vi "TypeDescriptor_ListElementNames.vi"(11 "type descriptor":i16[](array[numeric]) format="%04x") -> (1 "Has Elements":bool, 2 "element names":string[](array[string]), 3 "type descriptor dup":i16[](array[numeric]) format="%.0x", 4 "Event Class":string[](array[string]))   [LabVIEW 2013, in "OpenDescriptor.lvlib"]
uses:
  OpenDescriptor.lvlib
  TypeDescriptor_GetPString.vi
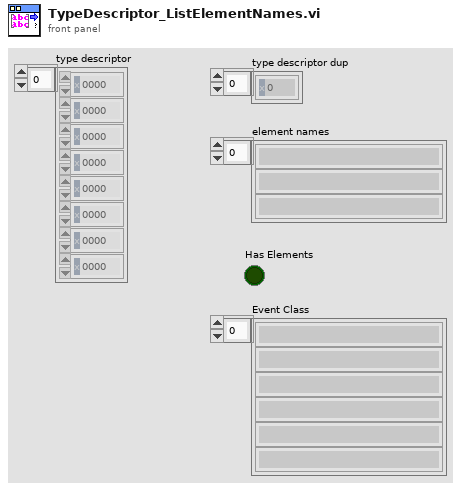
[diagram p1: front panel]
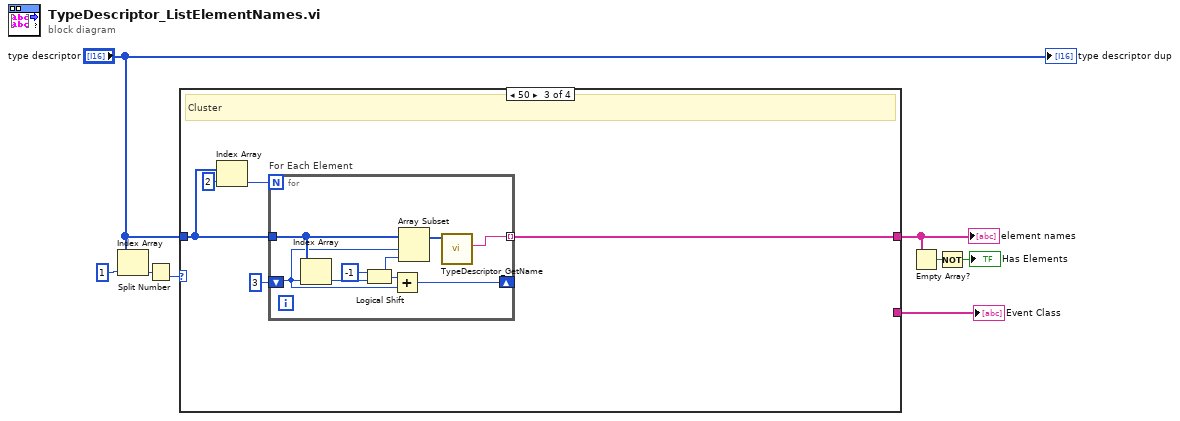
[diagram p0: block diagram]
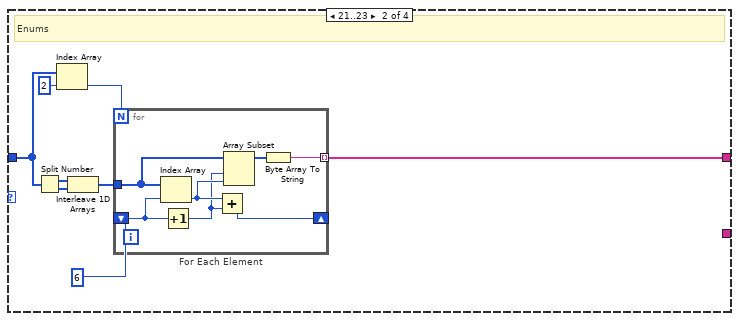
[diagram p3: hidden frame]
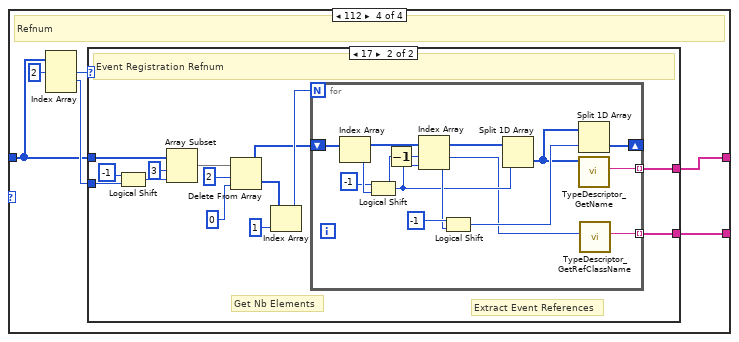
[diagram p4: hidden frame]
diagram:
  n1 = Index Array(array="type descriptor", index=1) -> (element=w8:i16)
  n2 = Split Number(x=w8) -> (lo(x)=w7:u8)  [unwired: 1 out]
  n3 = case shown="50" w7 {
    tunnel: [_ w9 w24 w38] -> w3
    tunnel: "type descriptor" -> [_ w10 w25 w39]
    tunnel: [_ _ _ w37] -> w1
    frame Default {
      # "This datatype is not a container or does not list elements"
    }
    frame 21..23 {
      # "Enums"
      n4 = Split Number(x=w10) -> (hi(x)=w13:u8[], lo(x)=w12:u8[])
      n5 = Index Array(array=w10, index=2) -> (element=w15:i16)
      n6 = Interleave 1D Arrays(w13, w12) -> (w11:u8[])
      n7 = for "For Each Element" {
        N: w15 -> [_]
        shift-right: [w20] -> _
        shift-left: 6 ("index") -> [w23]
        tunnel: w11 -> [w21]
        tunnel: [w18] -> w9 mode=indexing
        n8 = Index Array(array=w21, index=w23) -> (element=w19:u8)
        n9 = Increment(x=w23) -> (x+1=w17:i32)
        n10 = Add(x=w19, y=w17) -> (x+y=w20:i32)
        n11 = Array Subset(array=w21, index=w17, length=w19) -> (w22:u8[])
        n12 = Byte Array To String(unsigned byte array=w22) -> (string=w18:string)
      }
    }
    frame 80 {
      # "Cluster"
      n13 = Index Array(array=w25, index=2) -> (element=w27:i16)
      n14 = for "For Each Element" {
        N: w27 -> [_]
        tunnel: w25 -> [w33]
        shift-right: [w34] -> _
        shift-left: 3 ("index") -> [w32]
        tunnel: [w30] -> w24 mode=indexing
        n15 = Index Array(array=w33, index=w32) -> (element=w35:i16)
        n16 = Logical Shift(y=i16 -1, x=w35) -> (x << y=w31:i16)
        n17 = Add(x=w31, y=w32) -> (x+y=w34:i32)
        n18 = Array Subset(array=w33, index=w32, length=w31) -> (w29:i16[])
        n19 = call "TypeDescriptor_GetName.vi"("type descriptor"=w29) -> ("name"=w30:string)  [unwired: 8 in, 2 out]
      }
    }
    frame 112 {
      # "Refnum"
      n20 = Index Array(array=w39, index #1=2 ("index")) -> (element #1=w41:i16, element #2=w40:i16)  [unwired: 2 in, 1 out]
      n21 = case shown="17" w41 {
        tunnel: w40 -> [_ w53]
        tunnel: w39 -> [_ w56]
        tunnel: [_ w44] -> w38
        tunnel: [_ w43] -> w37
        frame 0, Default {
        }
        frame 23 {
          # "Extract Event References"
          # "Get Nb Elements"
          # "Event Registration Refnum"
          n22 = Logical Shift(y=i16 -1, x=w53) -> (x << y=w52:i16)
          n23 = Array Subset(array=w56, index=3, length=w52) -> (w51:i16[])
          n24 = Delete From Array(array=w51, length=2 ("index"), index=0) -> (deleted portion=w49:i16[], array with subset deleted=w45:i16[])
          n25 = Index Array(array=w49, index=1) -> (element=w46:i16)
          n26 = for {
            N: w46 -> [_]
            shift-right: [w59] -> _
            shift-left: w45 -> [w63]
            tunnel: [w64] -> w44 mode=indexing
            tunnel: [w57] -> w43 mode=indexing
            n27 = Index Array(array=w63) -> (element=w69:i16)  [unwired: 1 in]
            n28 = Logical Shift(y=i16 -1, x=w69) -> (x << y=w62:i16)
            n29 = Decrement(x=w62) -> (x-1=w65:i16)
            n30 = Index Array(array=w63, index #1=w65, index #2=w62) -> (element #1=w58:i16, element #2=w66:i16)
            n31 = Logical Shift(y=i16 -1, x=w66) -> (x << y=w61:i16)
            n32 = Split 1D Array(array=w63, index=w62) -> (second subarray=w60:i16[])  [unwired: 1 out]
            n33 = Split 1D Array(array=w60, index=w61) -> (second subarray=w59:i16[])  [unwired: 1 out]
            n34 = call "TypeDescriptor_GetName.vi"("type descriptor"=w60) -> ("name"=w64:string)  [unwired: 8 in, 2 out]
            n35 = call "TypeDescriptor_GetRefClassName.vi"("Ref Class"=w58) -> ("Reference Class"=w57:string)  [unwired: 10 in]
          }
        }
      }
    }
  }
  "element names" <- w3
  "Event Class" <- w1
  n36 = Empty Array?(array=w3) -> (empty?=w4:bool)
  n37 = Not(x=w4) -> (.not. x?=→"Has Elements":bool)
  "type descriptor dup" <- "type descriptor"
